vi "cluster2xml.vi"(8 "error in":errorcluster, 10 "Variant":variant, 11 "XML File Path":path) -> (0 "error out":errorcluster)   [LabVIEW 2013]
uses:
  <vilib>/NI/GXML/GXML.lvlib
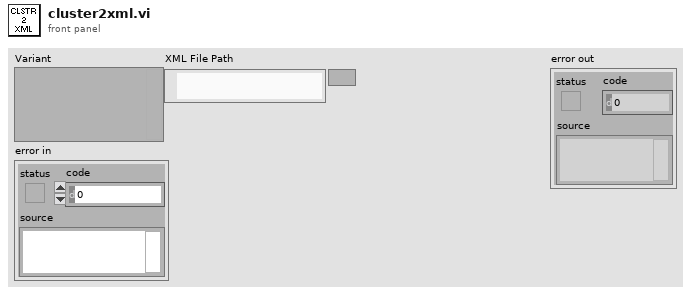
[diagram p1: front panel]
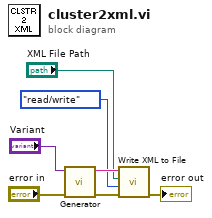
[diagram p0: block diagram]
diagram:
  n1 = call <vilib>:"Generator.vi"("error in"="error in", "Variant"="Variant") -> ("error out"=w5:errorcluster, "XML String Out"=w4:string)  [unwired: 8 in]
  n2 = call <vilib>:"Write XML to File.vi"("error in"=w5, "file access"=enum16{"read/write", "read-only", "write-only"}."read/write", "XML File Path"="XML File Path", "XML Input"=w4) -> ("error out"=→"error out":errorcluster)  [unwired: 7 in]
